vi "Move From Output to Export Dir.vi"(0 "NI Build Specification in":refnum<class "NIPKG_LV.lvclass">, 11 "error IO":errorcluster) -> (4 "NI Build Specification out":refnum<class "NIPKG_LV.lvclass">, 15 "error out":errorcluster)   [LabVIEW 2017, in "CL_G3_VIComponentBuilder.lvlib" / "NIPKG_LV.lvclass"]
doc: "Moves the NI Package from the Output Directory as defined by the NI Package build specification to the Component's export directory."
uses:
  NIPKG_LV.lvclass
  C:/builds/Component BuilderBT/SrcDist/Exports/Exports/Export.lvclass
  Exports/Export.lvclass/Export.ctl
  Exports/Accessors/Read Component Export Dir.vi
  Exports/Accessors/Read Exported Build Specification Path.vi
  Exports/Accessors/Write Built Export's Full Path.vi
  <vilib>/xml/Load XML File.vi
  <vilib>/xml/Close Reference(Node).vi
  <vilib>/Utility/file.llb/Is Path and Not Empty.vi
  <vilib>/Utility/error.llb/Error Cluster From Error Code.vi
  NI Build Specification_LV/NI Build Specification_LV.lvclass
  <vilib>/xml/NI_XML.lvlib
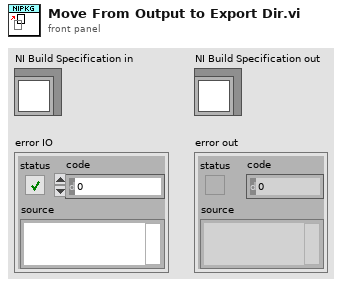
[diagram p1: front panel]
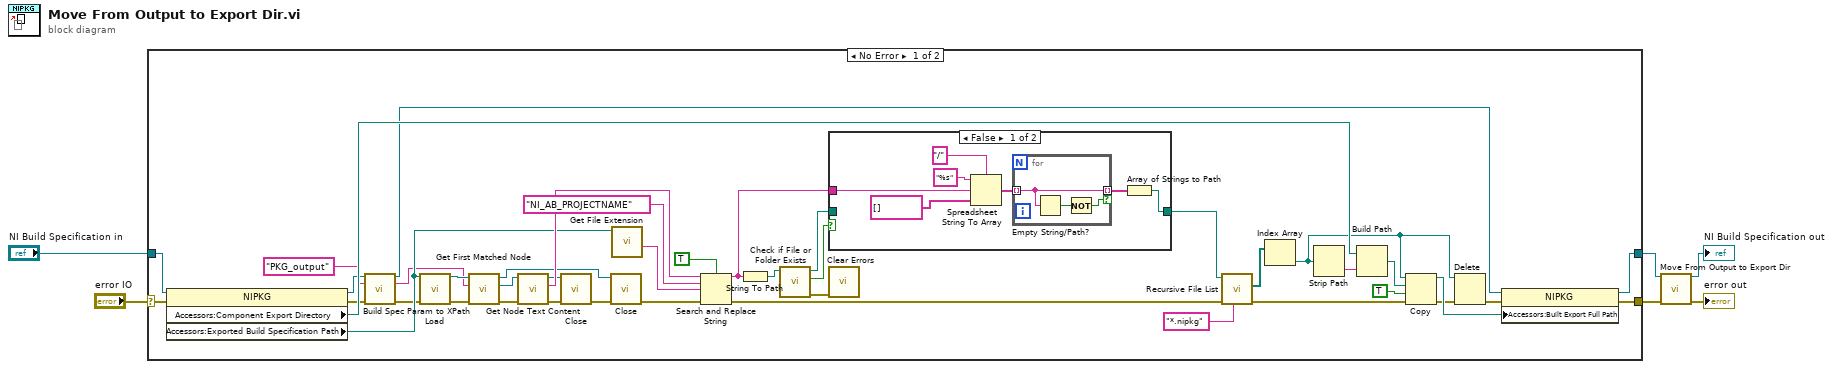
[diagram p0: block diagram]
diagram:
  n1 = case shown="No Error" "error IO" {
    selector: "error IO" -> [w45 w61]
    tunnel: [w44 w61] -> w4
    tunnel: "NI Build Specification in" -> [w46 w60]
    tunnel: [w21 w60] -> w3
    frame No Error {
      n2 = property class="NIPKG"(reference=w46, error in=w45) -> (reference out=w10:refnum<class "NIPKG_LV.lvclass">, error out=w12:errorcluster, "Accessors:Component Export Directory"=w25:path, "Accessors:Exported Build Specification Path"=w31:path)
      n3 = call-dynamic "Build Spec Param to XPath.vi"("NI Build Specification"=w10, "Build Spec Parameter Name"="PKG_output" ("input 4"), "error in (no error)"=w12) -> ("NI Build Specification"=w9:refnum<class "NIPKG_LV.lvclass">, "XPath to the specific build Spec Property"=w7:string, "error out"=w11:errorcluster)  [unwired: 10 in]
      n4 = call-poly <vilib>:"Load.vi"("path to XML document"=w31, "error in (no error)"=w11) -> ("DOM document out"=w38:refnum<k20>, "error out"=w39:errorcluster)  [unwired: 11 in, 1 out]
      n5 = call <vilib>:"Get First Matched Node.vi"("error in (no error)"=w39, "XPath expression"=w7, "node in"=w38) -> ("error out"=w35:errorcluster, "node result"=w34:refnum<k20>, "node out"=w36:refnum<k20>)  [unwired: 6 in]
      n6 = call <vilib>:"Get Node Text Content.vi"("error in (no error)"=w35, "node in"=w34) -> ("error out"=w37:errorcluster, "node text"=w42:string, "node out"=w41:refnum<k20>)  [unwired: 7 in]
      n7 = call-poly <vilib>:"Close.vi"("error in (no error)"=w37, "node"=w41) -> ("error out"=w40:errorcluster)  [unwired: 7 in]
      n8 = call-poly <vilib>:"Close.vi"("error in (no error)"=w40, "node"=w36) -> ("error out"=w30:errorcluster)  [unwired: 7 in]
      n9 = call <vilib>:"Get File Extension.vi"("file"=w31) -> ("filename without extension"=w43:string)  [unwired: 6 in, 4 out]
      n10 = Search and Replace String(case sensitive?=TRUE ("ignore case? (F)"), input string=w42, search string="NI_AB_PROJECTNAME", replace string=w43, error in=w30) -> (result string=w19:string, error out=w15:errorcluster)  [unwired: 3 in, 2 out]
      n11 = String To Path(string=w19) -> (path=w20:path)
      n12 = call <vilib>:"Check if File or Folder Exists.vi"("path"=w20) -> ("error out"=w16:errorcluster, "file or folder exists?"=w18:bool, "dup path"=w17:path)  [unwired: 8 in]
      n13 = case shown="False" w18 {
        tunnel: [w50 w59] -> w29
        tunnel: w19 -> [w49 _]
        tunnel: w17 -> [_ w59]
        frame False {
          n14 = Spreadsheet String To Array(delimiter (Tab)="/", format string="%s", spreadsheet string=w49, array type (2D Dbl)=string[] []) -> (array=w54:string[])
          n15 = for {
            tunnel: w54 -> [w57] mode=indexing
            tunnel: [w57] -> w55 mode=indexing if=w56
            n16 = Empty String/Path?(string/path=w57) -> (empty?=w58:bool)
            n17 = Not(x=w58) -> (.not. x?=w56:bool)
          }
          n18 = Array of Strings to Path(0:w55) -> (2:w50:path)  [unwired: 1 in]
        }
        frame True {
        }
      }
      n19 = call <vilib>:"Clear Errors.vi"("error in (no error)"=w16) -> ()  [unwired: 5 in, 2 out]
      n20 = call <vilib>:"Recursive File List.vi"("pattern"="*.nipkg", "error in (no error)"=w15, "Folder Path"=w29) -> ("error out"=w14:errorcluster, "All Files in Dir"=w27:path[])  [unwired: 4 in, 3 out]
      n21 = Index Array(array=w27) -> (element=w13:path)  [unwired: 1 in]
      n22 = Strip Path(path=w13) -> (name=w26:string)  [unwired: 1 out]
      n23 = Build Path(base path=w25, name or relative path=w26) -> (appended path=w24:path)
      n24 = Copy(8:w14, 9:TRUE ("overwrite (F)"), 10:w24, 11:w13) -> (0:w23:errorcluster, 3:w48:path)  [unwired: 1 in, 1 out]
      n25 = Delete(path (use dialog)=w13, error in=w23) -> (error out=w22:errorcluster)  [unwired: 3 in, 2 out]
      n26 = property class="NIPKG"(reference=w9, error in=w22, "Accessors:Built Export Full Path"=w48) -> (reference out=w21:refnum<class "NIPKG_LV.lvclass">, error out=w44:errorcluster)
    }
    frame Error {
    }
  }
  n27 = call-parent "Move From Output to Export Dir.vi"("NI Build Specification in"=w3, "error IO"=w4) -> ("NI Build Specification out"=→"NI Build Specification out":refnum<class "NIPKG_LV.lvclass">, "error out"=→"error out":errorcluster)  [unwired: 12 in]
